vi "sequencerGlobVars.vi"() -> ()   [LabVIEW 2014]
panel:
  in  "halt":bool
  in  "abort":bool
  in  "nOfScanRegions":i32
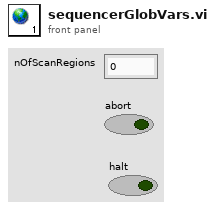
[diagram p1: front panel]
diagram:
